vi "loads_builder.vi"(7 "measure?":dbl, 8 "D / Y":bool, 9 "Carga mista":bool, 10 "Load (%/100)":string, 11 "Loads data":path) -> (3 "Loads (out)":string)   [LabVIEW 2020]
uses:
  <vilib>/Utility/file.llb/Read Delimited Spreadsheet (string).vi
panel:
  in  "X? ou L":bool=TRUE
  out "String":i32
  in  "Frequency (Hz)":dbl=50.0
  in  "Font (Vrms)":dbl=4160.0
  out "Powers":dbl[][](array[numeric])
  out "nós":dbl[](array[numeric])
  # "LOADS BUILDER"
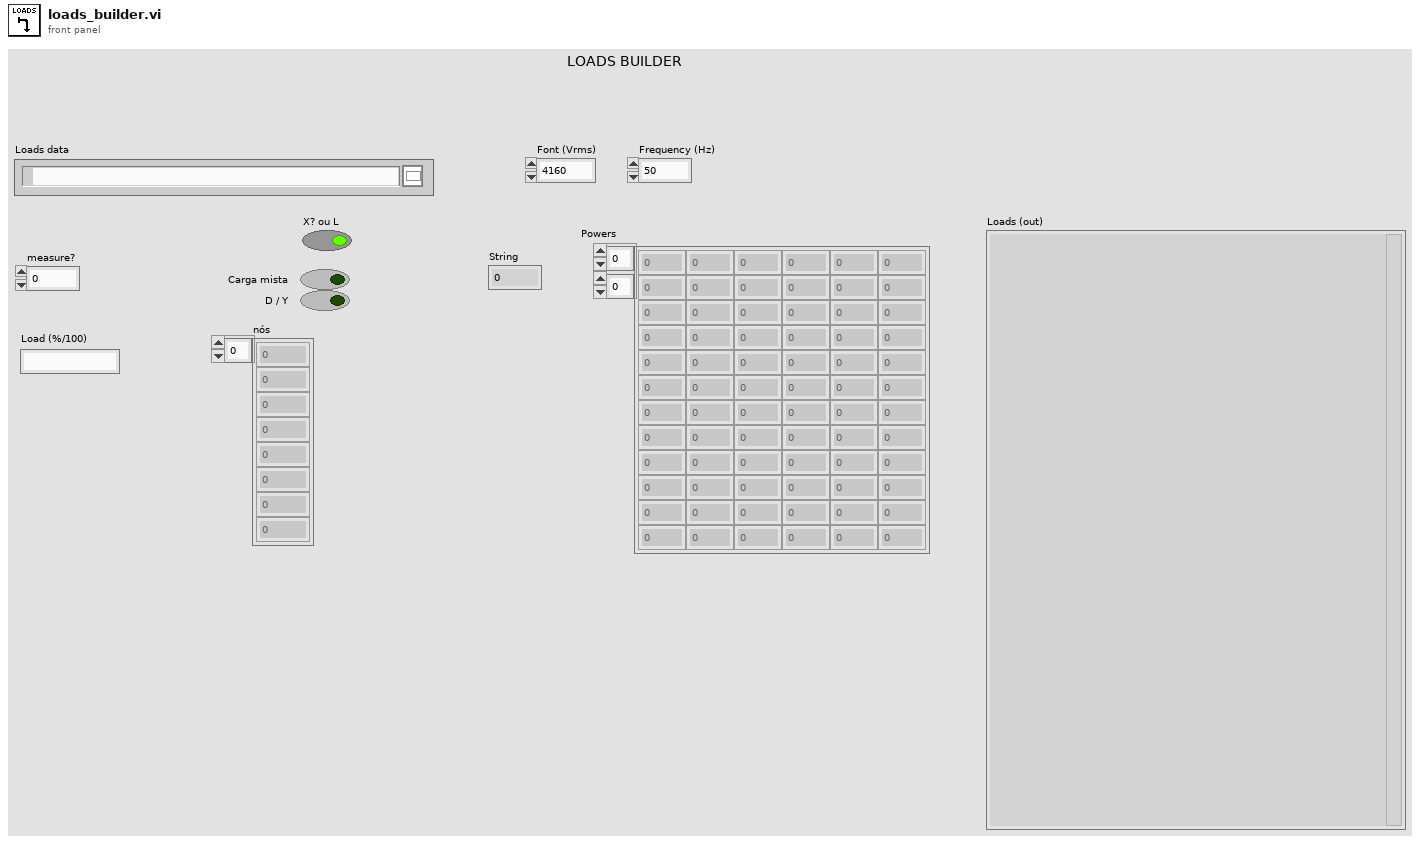
[diagram p1: front panel]
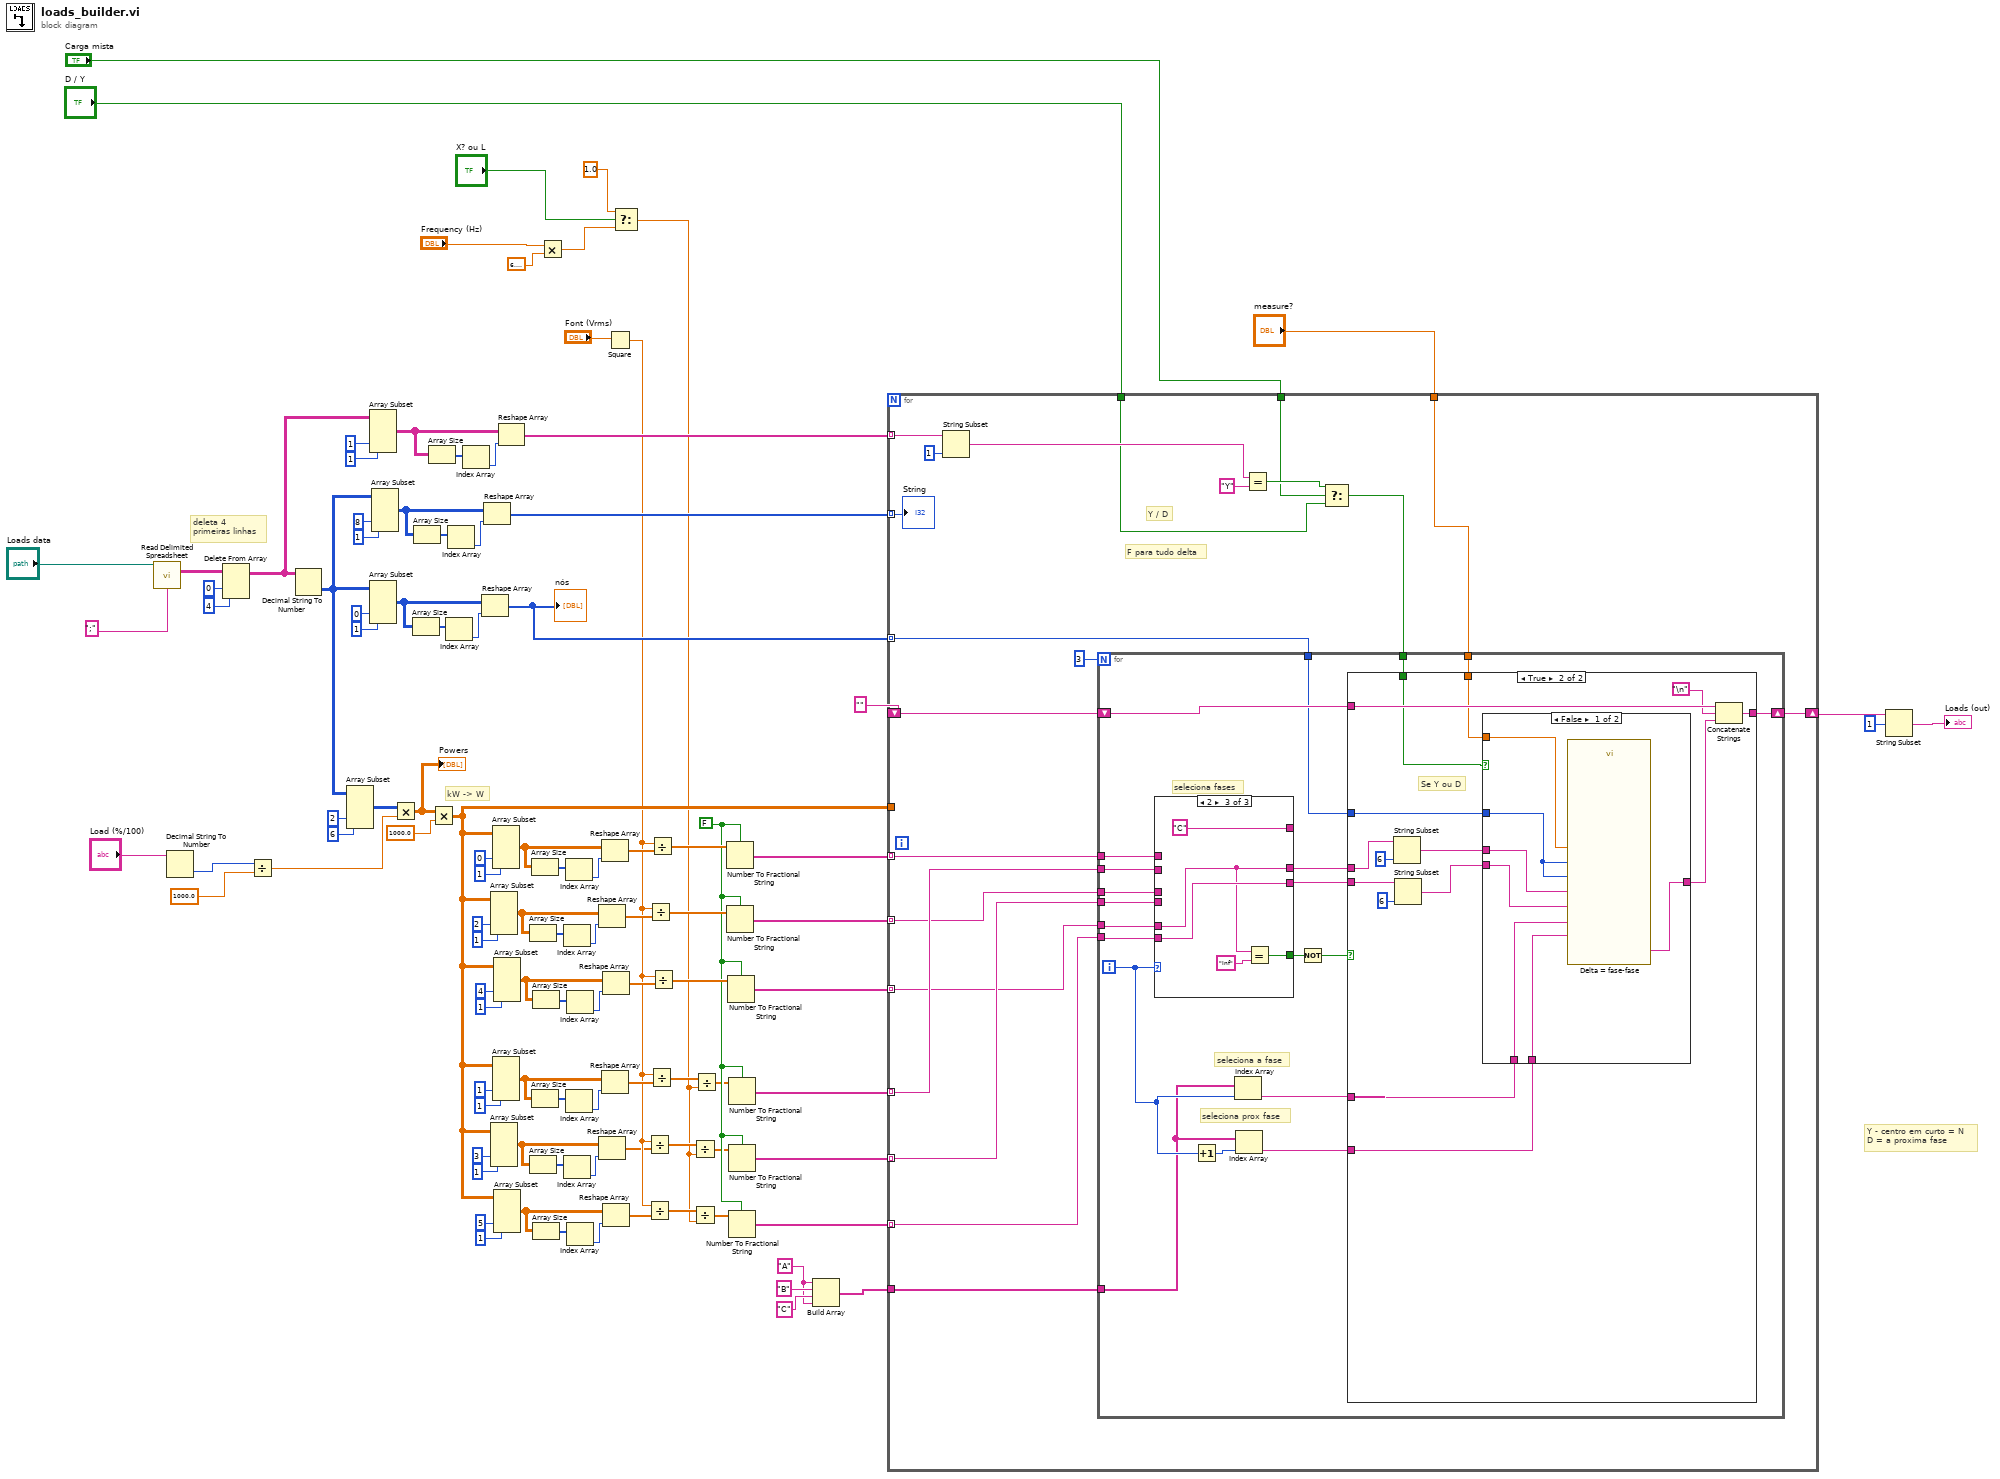
[diagram p0: block diagram]
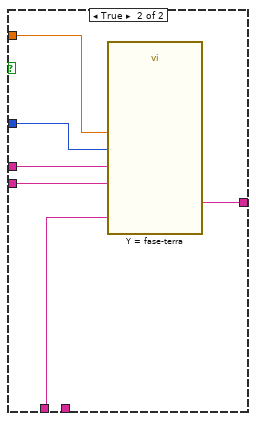
[diagram p3: hidden frame]
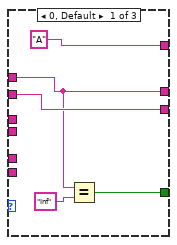
[diagram p4: hidden frame]
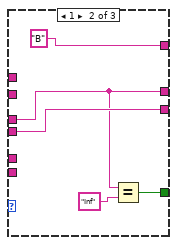
[diagram p5: hidden frame]
diagram:
  w7 = "A"
  w27 = FALSE ("use system decimal point (T)")
  # "Y - centro em curto = N\nD = a proxima fase"
  # "kW -> W"
  # "deleta 4\nprimeiras linhas"
  n1 = call-poly <vilib>:"Read Delimited Spreadsheet.vi"("file path (dialog if empty)"="Loads data", "delimiter (\\t)"=";" ("delimiter (\\t)")) -> ("all rows"=w77:string[][])  [unwired: 8 in, 5 out]
  n2 = Decimal String To Number(string="Load (%/100)") -> (number=w85:i32)  [unwired: 2 in, 1 out]
  n3 = Delete From Array(array=w77, length=4, index (row)=0) -> (array with subset deleted=w76:string[][])  [unwired: 1 in, 1 out]
  n4 = Divide(x=w85, y=1000.0) -> (x/y=w84:dbl)
  n5 = Decimal String To Number(string=w76) -> (number=w66:i32[][])  [unwired: 2 in, 1 out]
  n6 = Array Subset(array=w66, index (col)=2 ("index"), length (col)=6 ("length")) -> (w95:i32[][])  [unwired: 2 in]
  n7 = Array Subset(array=w76, index (col)=1 ("index"), length (col)=1 ("length")) -> (w73:string[][])  [unwired: 2 in]
  n8 = Array Subset(array=w66, index (col)=0 ("index"), length (col)=1 ("length")) -> (w104:i32[][])  [unwired: 2 in]
  n9 = Array Subset(array=w66, index (col)=8 ("index"), length (col)=1 ("length")) -> (w69:i32[][])  [unwired: 2 in]
  n10 = Multiply(x=w95, y=w84) -> (x*y=w88:dbl[][])
  "Powers" <- w88
  n11 = Array Size(array=w104) -> (size(s)=w103:i32[])
  n12 = Array Size(array=w69) -> (size(s)=w68:i32[])
  n13 = Array Size(array=w73) -> (size(s)=w75:i32[])
  n14 = Multiply(x=w88, y=1000.0) -> (x*y=w34:dbl[][])
  n15 = Index Array(array=w103) -> (element=w102:i32)  [unwired: 1 in]
  n16 = Index Array(array=w68) -> (element=w67:i32)  [unwired: 1 in]
  n17 = Index Array(array=w75) -> (element=w74:i32)  [unwired: 1 in]
  n18 = Reshape Array(w104, w102) -> (w101:i32[])
  "nós" <- w101
  n19 = Reshape Array(w69, w67) -> (w65:i32[])
  n20 = Array Subset(array=w34, index (col)=2 ("index"), length (col)=1 ("length")) -> (w55:dbl[][])  [unwired: 2 in]
  n21 = Array Subset(array=w34, index (col)=3 ("index"), length (col)=1 ("length")) -> (w40:dbl[][])  [unwired: 2 in]
  n22 = Array Subset(array=w34, index (col)=0 ("index"), length (col)=1 ("length")) -> (w60:dbl[][])  [unwired: 2 in]
  n23 = Array Subset(array=w34, index (col)=1 ("index"), length (col)=1 ("length")) -> (w45:dbl[][])  [unwired: 2 in]
  n24 = Array Subset(array=w34, index (col)=4 ("index"), length (col)=1 ("length")) -> (w50:dbl[][])  [unwired: 2 in]
  n25 = Array Subset(array=w34, index (col)=5 ("index"), length (col)=1 ("length")) -> (w35:dbl[][])  [unwired: 2 in]
  n26 = Reshape Array(w73, w74) -> (w72:string[])
  n27 = Array Size(array=w55) -> (size(s)=w57:i32[])
  n28 = Array Size(array=w40) -> (size(s)=w42:i32[])
  n29 = Array Size(array=w60) -> (size(s)=w62:i32[])
  n30 = Array Size(array=w45) -> (size(s)=w47:i32[])
  n31 = Array Size(array=w50) -> (size(s)=w52:i32[])
  n32 = Array Size(array=w35) -> (size(s)=w37:i32[])
  n33 = Multiply(x="Frequency (Hz)", y=6.283185307179586) -> (x*y=w4:dbl)
  n34 = Index Array(array=w57) -> (element=w56:i32)  [unwired: 1 in]
  n35 = Index Array(array=w42) -> (element=w41:i32)  [unwired: 1 in]
  n36 = Index Array(array=w62) -> (element=w61:i32)  [unwired: 1 in]
  n37 = Index Array(array=w47) -> (element=w46:i32)  [unwired: 1 in]
  n38 = Index Array(array=w52) -> (element=w51:i32)  [unwired: 1 in]
  n39 = Index Array(array=w37) -> (element=w36:i32)  [unwired: 1 in]
  n40 = Reshape Array(w55, w56) -> (w31:dbl[])
  n41 = Reshape Array(w40, w41) -> (w24:dbl[])
  n42 = Reshape Array(w60, w61) -> (w33:dbl[])
  n43 = Reshape Array(w45, w46) -> (w26:dbl[])
  n44 = Reshape Array(w50, w51) -> (w32:dbl[])
  n45 = Reshape Array(w35, w36) -> (w23:dbl[])
  n46 = Square(x="Font (Vrms)") -> (x^2=w25:dbl)
  n47 = Select(t=1.0, s="X? ou L", f=w4) -> (s? t:f=w3:dbl)
  n48 = Divide(x=w25, y=w24) -> (x/y=w21:dbl[])
  n49 = Divide(x=w25, y=w23) -> (x/y=w20:dbl[])
  n50 = Divide(x=w25, y=w31) -> (x/y=w29:dbl[])
  n51 = Divide(x=w25, y=w26) -> (x/y=w22:dbl[])
  n52 = Divide(x=w25, y=w33) -> (x/y=w30:dbl[])
  n53 = Divide(x=w25, y=w32) -> (x/y=w28:dbl[])
  n54 = Divide(x=w21, y=w3) -> (x/y=w18:dbl[])
  n55 = Divide(x=w20, y=w3) -> (x/y=w17:dbl[])
  n56 = Divide(x=w22, y=w3) -> (x/y=w19:dbl[])
  n57 = Number To Fractional String(use system decimal point (T)=w27, number=w30) -> (F-format string=w16:string[])  [unwired: 2 in]
  n58 = Number To Fractional String(use system decimal point (T)=w27, number=w29) -> (F-format string=w15:string[])  [unwired: 2 in]
  n59 = Number To Fractional String(use system decimal point (T)=w27, number=w28) -> (F-format string=w14:string[])  [unwired: 2 in]
  n60 = Number To Fractional String(use system decimal point (T)=w27, number=w19) -> (F-format string=w13:string[])  [unwired: 2 in]
  n61 = Number To Fractional String(use system decimal point (T)=w27, number=w18) -> (F-format string=w12:string[])  [unwired: 2 in]
  n62 = Number To Fractional String(use system decimal point (T)=w27, number=w17) -> (F-format string=w11:string[])  [unwired: 2 in]
  n63 = Build Array(w7, "B", "C", w7) -> (w8:string[])
  n64 = for {
    tunnel: w101 -> [w126] mode=indexing
    tunnel: w34 -> [_]
    shift-right: [w124] -> w93
    shift-left: "" -> [w125]
    tunnel: "measure?" -> [w123]
    tunnel: w72 -> [w122] mode=indexing
    tunnel: w65 -> [w120] mode=indexing
    tunnel: w16 -> [w119] mode=indexing
    tunnel: w15 -> [w117] mode=indexing
    tunnel: w14 -> [w115] mode=indexing
    tunnel: w13 -> [w118] mode=indexing
    tunnel: w12 -> [w116] mode=indexing
    tunnel: w11 -> [w114] mode=indexing
    tunnel: w8 -> [w113]
    tunnel: "Carga mista" -> [w109]
    tunnel: "D / Y" -> [w108]
    # "Y / D"
    # "F para tudo delta"
    n65 = String Subset(string=w122, length (rest)=1 ("length (rest)")) -> (substring=w112:string)  [unwired: 1 in]
    n66 = Equal?(x=w112, y="Y") -> (x = y?=w110:bool)
    n67 = Select(t=w110, s=w109, f=w108) -> (s? t:f=w107:bool)
    n68 = for {
      N: 3 -> [_]
      tunnel: w126 -> [w145]
      shift-right: [w146] -> w124
      shift-left: w125 -> [w147]
      tunnel: w123 -> [w144]
      tunnel: w119 -> [w143]
      tunnel: w118 -> [w142]
      tunnel: w117 -> [w139]
      tunnel: w116 -> [w138]
      tunnel: w115 -> [w137]
      tunnel: w114 -> [w136]
      tunnel: w113 -> [w130]
      tunnel: w107 -> [w128]
      i -> [w131]
      # "seleciona prox fase"
      # "seleciona a fase"
      # "seleciona fases"
      n69 = case shown="2" w131 {
        tunnel: ["A" "B" "C"] -> _
        tunnel: w143 -> [w178 _ _]
        tunnel: w142 -> [w180 _ _]
        tunnel: [w178 w183 w188] -> w141
        tunnel: [w180 w185 w190] -> w140
        tunnel: w139 -> [_ w183 _]
        tunnel: w138 -> [_ w185 _]
        tunnel: w137 -> [_ _ w188]
        tunnel: w136 -> [_ _ w190]
        tunnel: [w177 w182 w187] -> w135
        frame 0, Default {
          n70 = Equal?(x=w178, y="Inf") -> (x = y?=w177:bool)
        }
        frame 1 {
          n71 = Equal?(x=w183, y="Inf") -> (x = y?=w182:bool)
        }
        frame 2 {
          n72 = Equal?(x=w188, y="Inf") -> (x = y?=w187:bool)
        }
      }
      n73 = Increment(x=w131) -> (x+1=w132:i32)
      n74 = Index Array(array=w130, index=w131) -> (element=w133:string)
      n75 = Index Array(array=w130, index=w132) -> (element=w129:string)
      n76 = Not(x=w135) -> (.not. x?=w134:bool)
      n77 = case shown="True" w134 {
        tunnel: w147 -> [w148 w163]
        tunnel: [w148 w160] -> w146
        tunnel: w140 -> [_ w155]
        tunnel: w141 -> [_ w157]
        tunnel: w133 -> [_ w153]
        tunnel: w145 -> [_ w154]
        tunnel: w144 -> [_ w159]
        tunnel: w129 -> [_ w150]
        tunnel: w128 -> [_ w149]
        frame False {
        }
        frame True {
          # "Se Y ou D"
          n78 = String Subset(string=w157, length (rest)=6 ("length (rest)")) -> (substring=w152:string)  [unwired: 1 in]
          n79 = String Subset(string=w155, length (rest)=6 ("length (rest)")) -> (substring=w151:string)  [unwired: 1 in]
          n80 = case shown="False" w149 {
            tunnel: [w170 w176] -> w161
            tunnel: w159 -> [w169 w175]
            tunnel: w154 -> [w168 w174]
            tunnel: w153 -> [w165 w173]
            tunnel: w152 -> [w167 w172]
            tunnel: w151 -> [w166 w171]
            tunnel: w150 -> [w164 _]
            frame False {
              n81 = call "Delta = fase-fase"("fase_out"=w164, "reatancia"=w166, "no_in"=w168, "fase_in"=w165, "no_out"=w168, "resistencia"=w167, "measure"=w169) -> ("Result"=w170:string)  [unwired: 7 in, 1 out]
            }
            frame True {
              n82 = call "Y = fase-terra"("reatancia"=w171, "no"=w174, "fase"=w173, "resistencia"=w172, "measure"=w175) -> ("Result"=w176:string)  [unwired: 9 in, 1 out]
            }
          }
          n83 = Concatenate Strings(w163, "\n", w161) -> (w160:string)
        }
      }
    }
    "String" <- w120
  }
  n84 = String Subset(string=w93, offset (0)=1) -> (substring=→"Loads (out)":string)  [unwired: 1 in]
